vi "VIG - Element DB.vi"(0 "Tree Ref In":refnum<vi>, 5 "Element Tag":string, 7 "Tree Element Data In":variant, 11 "error in (no error)":errorcluster, 13 "Command":T1) -> (2 "replaced":bool, 3 "Found":bool, 4 "Tree Ref Out":refnum<vi>, 6 "Element Tag Out":string, 8 "Tree Element Data Out":variant, 15 "error out":errorcluster)   [LabVIEW 2012, in "QuickVIew.lvlib"]
uses:
  QuickVIew.lvlib
  Typedef/TYPEDEF - DataStore Command.ctl
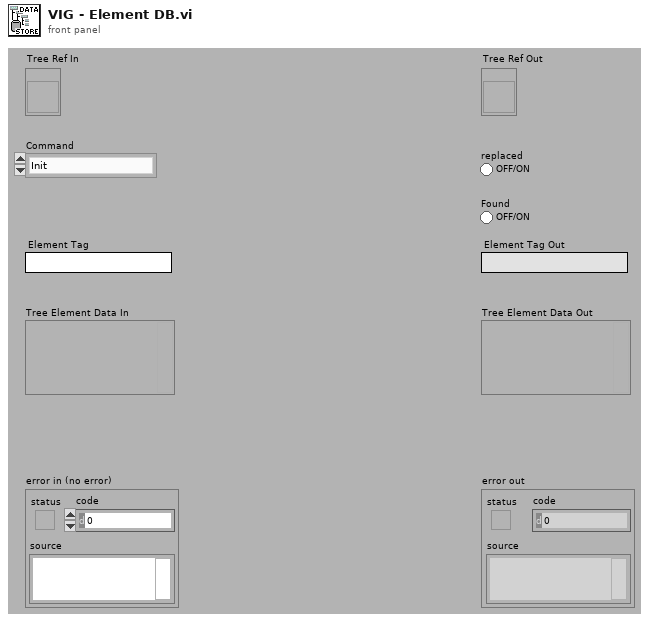
[diagram p1: front panel]
types:
  T1 = typedef "QuickVIew.lvlib/TYPEDEF - DataStore Command.ctl" = enum16{"Init", "Add", "Get", "Clear Tree", "Clear All", "Modify"}
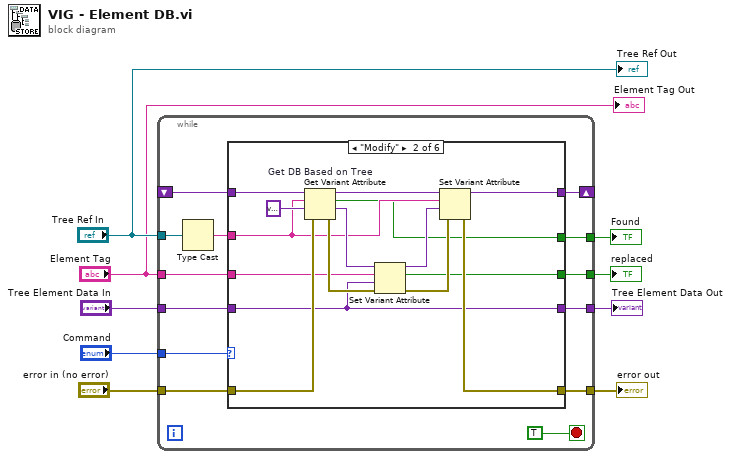
[diagram p0: block diagram]
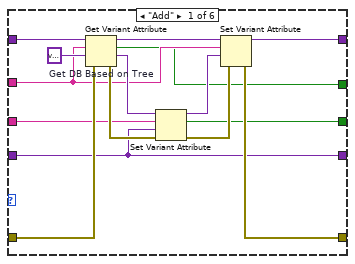
[diagram p2: hidden frame]
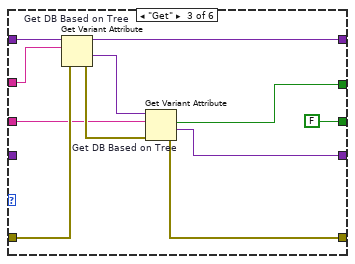
[diagram p3: hidden frame]
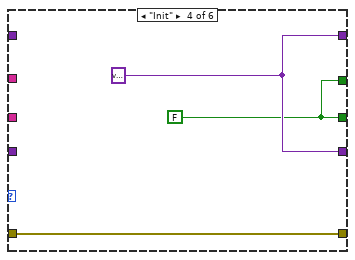
[diagram p4: hidden frame]
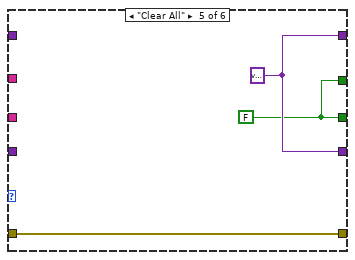
[diagram p5: hidden frame]
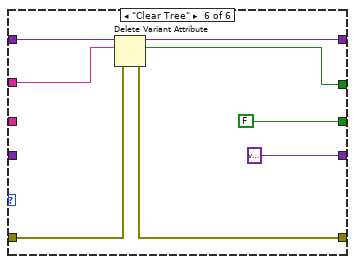
[diagram p6: hidden frame]
diagram:
  n1 = while {
    tunnel: "Tree Ref In" -> [w13]
    tunnel: "Command" -> [w21]
    tunnel: "Tree Element Data In" -> [w20]
    shift-right: [w19] -> _
    shift-left: _ -> [w18]
    tunnel: "Element Tag" -> [w17]
    tunnel: "error in (no error)" -> [w16]
    tunnel: [w15] -> w5
    tunnel: [w14] -> w4
    tunnel: [w11] -> w3
    tunnel: [w10] -> w2
    stop <- TRUE stop-if-true
    n2 = Type Cast(x=w13) -> (*(type *) &x=w12:string)  [unwired: 1 out]
    n3 = case shown="\"Modify\"" w21 {
      tunnel: w20 -> [w24 w39 _ _ _ _]
      tunnel: [w27 w42 w55 w65 w68 w75] -> w19
      tunnel: w18 -> [w33 w48 w62 _ _ w77]
      tunnel: w17 -> [w30 w45 w58 _ _ _]
      tunnel: w16 -> [w35 w50 w60 w66 w69 w72]
      tunnel: [w36 w51 w56 w66 w69 w73] -> w15
      tunnel: [w29 w44 FALSE ("replaced") w64 w67 FALSE ("replaced")] -> w14
      tunnel: w12 -> [w25 w40 w61 _ _ w76]
      tunnel: [w24 w39 w57 w65 w68 variant ("Tree Element Data 2")] -> w11
      tunnel: [w23 w38 w53 w64 w67 w71] -> w10
      frame "Add" {
        n4 = Get Variant Attribute "Get DB Based on Tree"(Variant=w33, name=w25, default value (empty Variant)=variant ("default value (empty variant)"), error in=w35) -> (duplicate Variant=w28:variant, found=w23:bool, value=w31:variant, error out=w34:errorcluster)
        n5 = Set Variant Attribute(Variant=w31, name=w30, value=w24, error in=w34) -> (Variant out=w26:variant, replaced=w29:bool, error out=w37:errorcluster)
        n6 = Set Variant Attribute(Variant=w28, name=w25, value=w26, error in=w37) -> (Variant out=w27:variant, error out=w36:errorcluster)  [unwired: 1 out]
      }
      frame "Modify" {
        n7 = Get Variant Attribute "Get DB Based on Tree"(Variant=w48, name=w40, default value (empty Variant)=variant ("default value (empty variant)"), error in=w50) -> (duplicate Variant=w43:variant, found=w38:bool, value=w46:variant, error out=w49:errorcluster)
        n8 = Set Variant Attribute(Variant=w46, name=w45, value=w39, error in=w49) -> (Variant out=w41:variant, replaced=w44:bool, error out=w52:errorcluster)
        n9 = Set Variant Attribute(Variant=w43, name=w40, value=w41, error in=w52) -> (Variant out=w42:variant, error out=w51:errorcluster)  [unwired: 1 out]
      }
      frame "Get" {
        n10 = Get Variant Attribute "Get DB Based on Tree"(Variant=w62, name=w61, error in=w60) -> (duplicate Variant=w55:variant, value=w59:variant, error out=w63:errorcluster)  [unwired: 1 in, 1 out]
        n11 = Get Variant Attribute "Get DB Based on Tree"(Variant=w59, name=w58, error in=w63) -> (found=w53:bool, value=w57:variant, error out=w56:errorcluster)  [unwired: 1 in, 1 out]
      }
      frame "Init" {
        w64 = FALSE ("replaced")
        w65 = variant ("Tree Element Data 2")
      }
      frame "Clear All" {
        w67 = FALSE ("replaced")
        w68 = variant ("Tree Element Data 2")
      }
      frame "Clear Tree" {
        n12 = Delete Variant Attribute(4:w72, 6:w76, 7:w77) -> (0:w73:errorcluster, 2:w71:bool, 3:w75:variant)
      }
    }
  }
  "error out" <- w5
  "replaced" <- w4
  "Tree Element Data Out" <- w3
  "Found" <- w2
  "Tree Ref Out" <- "Tree Ref In"
  "Element Tag Out" <- "Element Tag"
